vi "Test - Inversor - Set Voltage 1.vi"(8 "error in":errorcluster, 10 "Voltage":dbl, 11 "Module ID":i32) -> (0 "error out":errorcluster, 3 "Command":string)   [LabVIEW 2019]
doc: "_____\nCreated using DQMH Framework: Event Scripter 7.1.0.1503."
uses:
  Libraries/Inversor/Inversor.lvlib
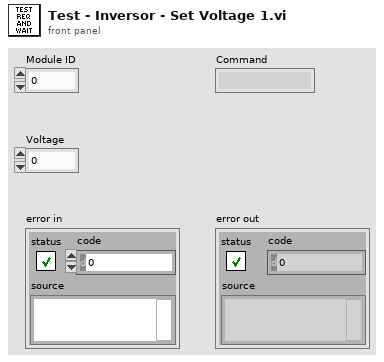
[diagram p1: front panel]
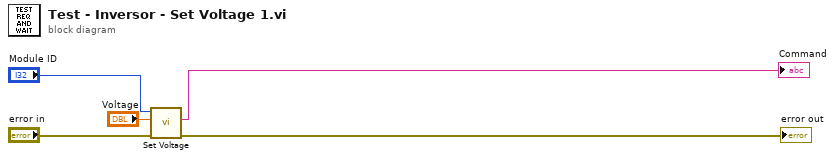
[diagram p0: block diagram]
diagram:
  n1 = call "Set Voltage.vi"("error in"="error in", "Voltage"="Voltage", "Module ID"="Module ID") -> ("error out"=→"error out":errorcluster, "Command"=→"Command":string)  [unwired: 6 in, 1 out]
